vi "MessageBase.setFieldSpecByName.vi"(8 "error in (no error)":errorcluster, 9 "FIeldSpec":T1, 10 "Field.Name":string="Canceled Quantity", 11 "MessageBase in":refnum<class "MessageBase.lvclass">) -> (0 "error out":errorcluster, 3 "MessageBase out":refnum<class "MessageBase.lvclass">)   [LabVIEW 2022 SP3, in "MessageBase.lvclass"]
uses:
  MessageBase.lvclass
  FieldSpec.ctl
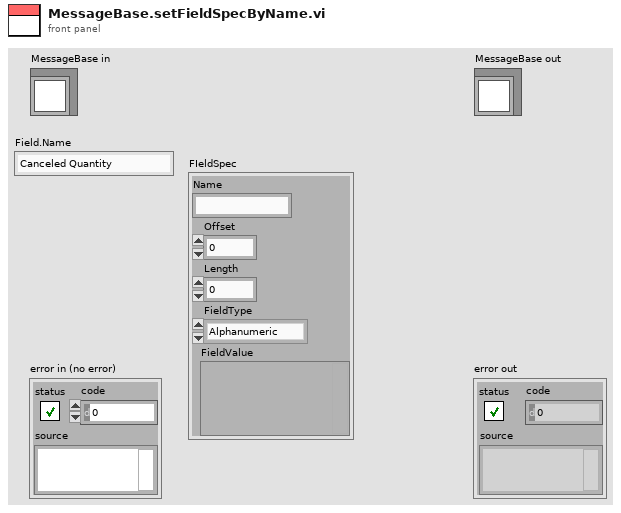
[diagram p1: front panel]
types:
  T1 = typedef "FieldSpec.ctl" = cluster{"Name":string, "Offset":i32, "Length":i32, "FieldType":enum16{"Alphanumeric", "Binary", "BinaryLongPrice", "BinaryShortPrice", "BitField", "PrintableAscii", "Value"}, "FieldValue":variant}
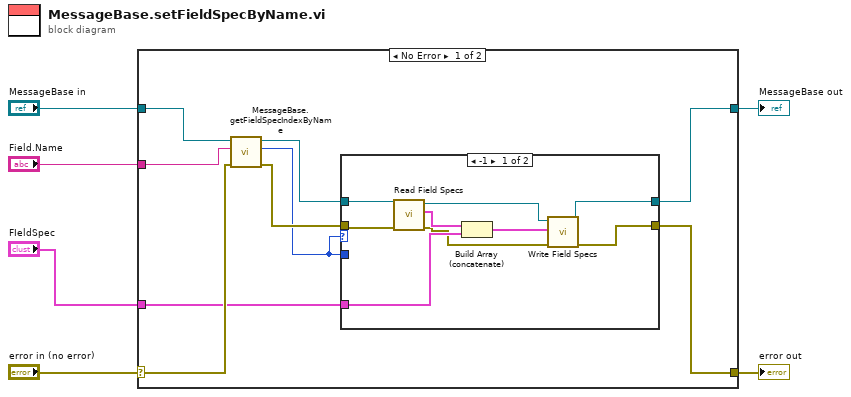
[diagram p0: block diagram]
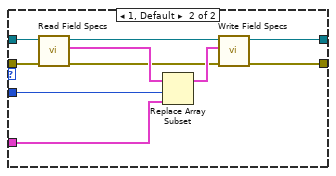
[diagram p2: hidden frame]
diagram:
  n1 = case shown="No Error" "error in (no error)" {
    selector: "error in (no error)" -> [w11 w36]
    tunnel: [w9 w36] -> w5
    tunnel: [w8 w35] -> w3
    tunnel: "MessageBase in" -> [w14 w35]
    tunnel: "Field.Name" -> [w15 _]
    tunnel: "FIeldSpec" -> [w10 _]
    frame No Error {
      n2 = call-dynamic "MessageBase.getFieldSpecIndexByName.vi"("error in (no error)"=w11, "Field.Name"=w15, "MessageBase in"=w14) -> ("error out"=w12:errorcluster, "Index"=w7:i32, "MessageBase out"=w13:refnum<class "MessageBase.lvclass">)  [unwired: 6 in]
      n3 = case shown="-1" w7 {
        tunnel: w13 -> [w24 w30]
        tunnel: w12 -> [w23 w29]
        tunnel: w7 -> [_ w28]
        tunnel: w10 -> [w21 w27]
        tunnel: [w17 w26] -> w9
        tunnel: [w16 w25] -> w8
        frame -1 {
          n4 = call-dynamic "Read Field Specs.vi"("error in (no error)"=w23, "MessageBase in"=w24) -> ("error out"=w18:errorcluster, "Field Specs"=w22:T1[], "MessageBase out"=w19:refnum<class "MessageBase.lvclass">)  [unwired: 7 in]
          n5 = Build Array (concatenate)(w22, w21) -> (w20:T1[])
          n6 = call-dynamic "Write Field Specs.vi"("error in (no error)"=w18, "Field Specs"=w20, "MessageBase in"=w19) -> ("error out"=w17:errorcluster, "MessageBase out"=w16:refnum<class "MessageBase.lvclass">)  [unwired: 7 in]
        }
        frame 1, Default {
          n7 = call-dynamic "Read Field Specs.vi"("error in (no error)"=w29, "MessageBase in"=w30) -> ("error out"=w31:errorcluster, "Field Specs"=w33:T1[], "MessageBase out"=w34:refnum<class "MessageBase.lvclass">)  [unwired: 7 in]
          n8 = Replace Array Subset(array=w33, new element=w27, index=w28) -> (w32:T1[])
          n9 = call-dynamic "Write Field Specs.vi"("error in (no error)"=w31, "Field Specs"=w32, "MessageBase in"=w34) -> ("error out"=w26:errorcluster, "MessageBase out"=w25:refnum<class "MessageBase.lvclass">)  [unwired: 7 in]
        }
      }
    }
    frame Error {
    }
  }
  "error out" <- w5
  "MessageBase out" <- w3
